vi "LCDIO Lookup In Chan By Name.vi"(8 "error in (no error)":errorcluster caption="Fehler (Eingang, kein Fehler)", 11 "Input Channel Name":string) -> (0 "error out":errorcluster caption="Fehler (Ausgang)", 3 "Input Channel Handle":i64)   [LabVIEW 2021, in "labbCAN_DigIO_API.lvlib"]
doc: "LCDIO_Func long LCDIO_CALL LCDIO_LookupInChanByName(const char* pChannelName,\n dev_hdl* pInChanHdl);"
uses:
  labbCAN_DigIO_API.lvlib
  labbCAN_DigIO_API.dll
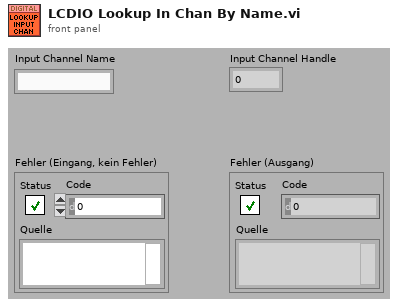
[diagram p1: front panel]
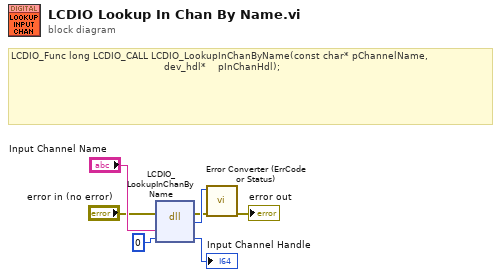
[diagram p0: block diagram]
diagram:
  # "LCDIO_Func long LCDIO_CALL LCDIO_LookupInChanByName(const char* pChannelName,\n                                                   dev_hdl*    pInChanHdl);"
  n1 = dll-call lib="C:/Users/olaja/AppData/Local/CETONI_SDK/labbCAN_DigIO_API.*" fn="LCDIO_LookupInChanByName"(error in="error in (no error)", "Input Channel Name"="Input Channel Name", "Input Channel Handle"=i64 0) -> (error out=w2:errorcluster, "Rückgabetyp"=w3:i32, "Input Channel Handle"=→"Input Channel Handle":i64)  [unwired: 3 in, 1 out]
  n2 = call "Error Converter (ErrCode or Status).vi"("error in (no error)"=w2, "error code"=w3) -> ("error out"=→"error out":errorcluster)  [unwired: 9 in]
